vi "Console.vi"(8 "error in (no error)":errorcluster caption="错误输入（无错误）", 9 "Mode":enum16{"Write", "Read", "Clear"}(ring)=enum."Clear", 11 "Input":string) -> (0 "error out":errorcluster caption="错误输出", 3 "Output":string)   [LabVIEW 2013]
doc: "该模板用于创建子VI。"
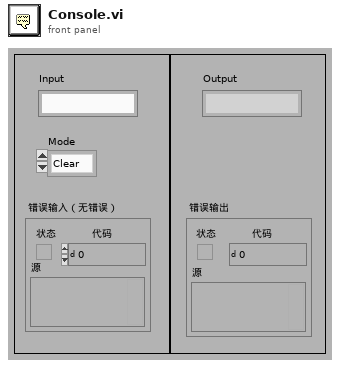
[diagram p1: front panel]
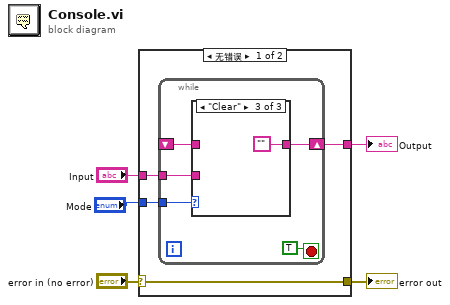
[diagram p0: block diagram]
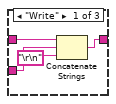
[diagram p2: hidden frame]
diagram:
  n1 = case shown="无错误" "error in (no error)" {
    selector: "error in (no error)" -> [w7 w21]
    tunnel: [w7 w21] -> w4
    tunnel: "Mode" -> [w9 _]
    tunnel: "Input" -> [w8 _]
    tunnel: [w6 _] -> w1
    frame No Error {
      n2 = while {
        tunnel: w9 -> [w13]
        shift-right: [w12] -> w6
        shift-left: _ -> [w11]
        tunnel: w8 -> [w10]
        stop <- TRUE stop-if-true
        n3 = case shown="\"Clear\"" w13 {
          tunnel: [w15 w19 ""] -> w12
          tunnel: w11 -> [w18 w19 _]
          tunnel: w10 -> [w17 _ _]
          frame "Write" {
            n4 = Concatenate Strings(w18, w17, "\r\n") -> (w15:string)
          }
          frame "Read", Default {
          }
          frame "Clear" {
          }
        }
      }
    }
    frame Error {
    }
  }
  "error out" <- w4
  "Output" <- w1
